vi "Obtain Request Events.vi"(8 "error in (no error)":errorcluster, 10 "Create New? (F)":bool) -> (0 "error out":errorcluster, 2 "Panther Dashboard Request Events":T1)   [LabVIEW 2023, in "Panther Dashboard.lvlib"]
doc: "This VI Obtains/Creates the Requests events that will be used for other modules to communicate with the module that owns this VI. These Requests events will be accessed only via Public API methods for this module.\n\n<b>NOTE</b>: The contents of this VI are automatically generated and modified by the <b>Tools > Delacor > DQMH</b> utilities. Consider using those utilities instead of making your own modifications to this VI.\n_____\nBased on DQMH Project Template 6.1.0.94."
uses:
  Panther Dashboard.lvlib
  Request Events--cluster.ctl
  Stop Argument--cluster.ctl
  Show Panel Argument--cluster.ctl
  Hide Panel Argument--cluster.ctl
  Get Module Execution Status Argument--cluster.ctl
  Show Diagram Argument--cluster.ctl
  Scan DQMH Modules Argument--cluster.ctl
  Tree DQMH Selection Argument--cluster.ctl
  Open Module API Tester Argument--cluster.ctl
  Execute Default Event Request Argument--cluster.ctl
  Expand Results Argument--cluster.ctl
  Launch DQMH Scripting Tools Argument--cluster.ctl
  DQMH Tools Menu--enum.ctl
  Generate Project Documentation Argument--cluster.ctl
  Set App Theme Argument--cluster.ctl
  Show About Argument--cluster.ctl
  Update Module ID Argument--cluster.ctl
  Save Library Description Argument--cluster.ctl
  Save VI Description Argument--cluster.ctl
  Open Documentation Argument--cluster.ctl
  Save Project Documentation Argument--cluster.ctl
  Register controls Mouse Enter Argument--cluster.ctl
  Save Module Spec Argument--cluster.ctl
panel:
  # "NOTE: The contents of this VI are automatically generated and modified by the Tools > Delacor > DQMH utilities. Consider using those utilities instead of making your own modifications to this VI."
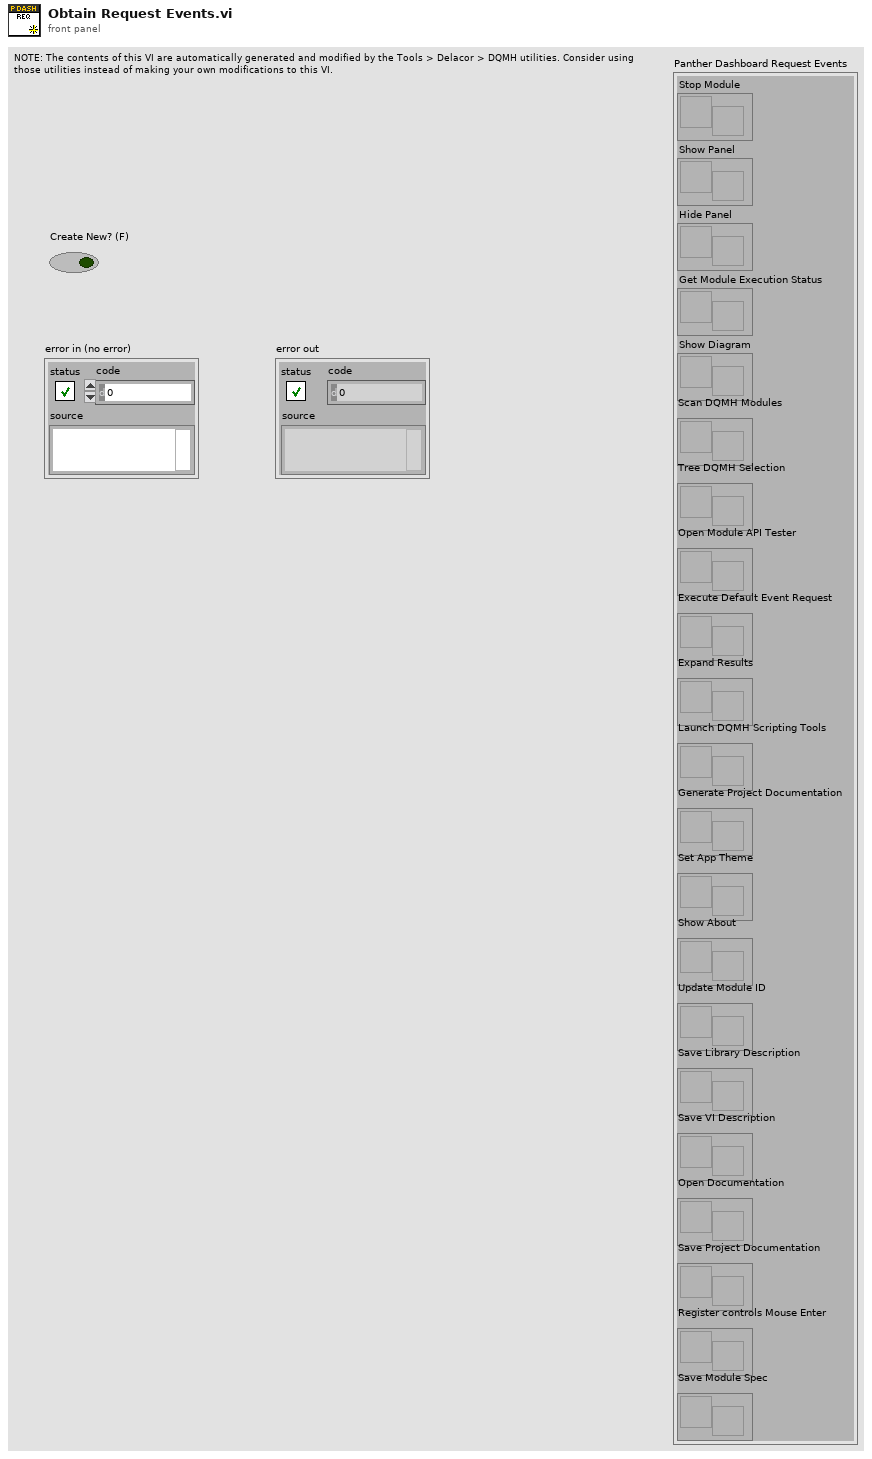
[diagram p1: front panel]
types:
  T1 = typedef "Panther Dashboard.lvlib/Request Events--cluster.ctl" = cluster{"Stop Module":refnum<user-event>, "Show Panel":refnum<user-event>, "Hide Panel":refnum<user-event>, "Get Module Execution Status":refnum<user-event>, "Show Diagram":refnum<user-event>, "Scan DQMH Modules":refnum<user-event>, "Tree DQMH Selection":refnum<user-event>, "Open Module API Tester":refnum<user-event>, "Execute Default Event Request":refnum<user-event>, "Expand Results":refnum<user-event>, "Launch DQMH Scripting Tools":refnum<user-event>, "Generate Project Documentation":refnum<user-event>, "Set App Theme":refnum<user-event>, "Show About":refnum<user-event>, "Update Module ID":refnum<user-event>, "Save Library Description":refnum<user-event>, "Save VI Description":refnum<user-event>, "Open Documentation":refnum<user-event>, "Save Project Documentation":refnum<user-event>, "Register controls Mouse Enter":refnum<user-event>, "Save Module Spec":refnum<user-event>}
  T2 = typedef "Panther Dashboard.lvlib/Save Module Spec Argument--cluster.ctl" = cluster{"Boolean":bool}
  T3 = typedef "Panther Dashboard.lvlib/Register controls Mouse Enter Argument--cluster.ctl" = cluster{"Boolean":bool}
  T4 = typedef "Panther Dashboard.lvlib/Save Project Documentation Argument--cluster.ctl" = cluster{"Project Description":string}
  T5 = typedef "Panther Dashboard.lvlib/Open Documentation Argument--cluster.ctl" = cluster{"Boolean":bool}
  T6 = typedef "Panther Dashboard.lvlib/Save VI Description Argument--cluster.ctl" = cluster{"VI Description":string}
  T7 = typedef "Panther Dashboard.lvlib/Save Library Description Argument--cluster.ctl" = cluster{"Library Description":string}
  T8 = typedef "Panther Dashboard.lvlib/Update Module ID Argument--cluster.ctl" = cluster{"New ID":i32}
  T9 = typedef "Panther Dashboard.lvlib/Show About Argument--cluster.ctl" = cluster{"Boolean":bool}
  T10 = typedef "Panther Dashboard.lvlib/Set App Theme Argument--cluster.ctl" = cluster{"Theme":bool}
  T11 = typedef "Panther Dashboard.lvlib/Generate Project Documentation Argument--cluster.ctl" = cluster{"Boolean":bool}
  T12 = typedef "Panther Dashboard.lvlib/Launch DQMH Scripting Tools Argument--cluster.ctl" = cluster{"Scripting Tool":T13}
  T13 = typedef "Panther Dashboard.lvlib/DQMH Tools Menu--enum.ctl" = enum16{"Create New DQMH Event", "Remove DQMH Event", "Convert DQMH Event", "Rename DQMH Event", "Add New DQMH Module", "Create RT Tester", "Rename DQMH Module", "Validate DQMH Module", "Create DQMH Module Template", "New DQMH  Unit Test", "Add Helper Loop to DQMH Module"}
  T14 = typedef "Panther Dashboard.lvlib/Expand Results Argument--cluster.ctl" = cluster{"Expand?":bool}
  T15 = typedef "Panther Dashboard.lvlib/Execute Default Event Request Argument--cluster.ctl" = cluster{"Event Name":string}
  T16 = typedef "Panther Dashboard.lvlib/Open Module API Tester Argument--cluster.ctl" = cluster{"Boolean":bool}
  T17 = typedef "Panther Dashboard.lvlib/Tree DQMH Selection Argument--cluster.ctl" = cluster{"Tree DQMH Sel":string}
  T18 = typedef "Panther Dashboard.lvlib/Scan DQMH Modules Argument--cluster.ctl" = cluster{"Include Dependencies":bool, "Scan All":bool, "Project":string, "Target":string}
  T19 = typedef "Panther Dashboard.lvlib/Hide Panel Argument--cluster.ctl" = cluster{"Hide Panel?":bool}
  T20 = typedef "Panther Dashboard.lvlib/Show Panel Argument--cluster.ctl" = cluster{"Show Panel?":bool}
  T21 = typedef "Panther Dashboard.lvlib/Show Diagram Argument--cluster.ctl" = cluster{"Debug?":bool}
  T22 = typedef "Panther Dashboard.lvlib/Get Module Execution Status Argument--cluster.ctl" = cluster{"Running?":bool}
  T23 = typedef "Panther Dashboard.lvlib/Stop Argument--cluster.ctl" = cluster{"Origin":string, "Exit via Stop Module Req?":bool, "Wait for Module to stop?":bool}
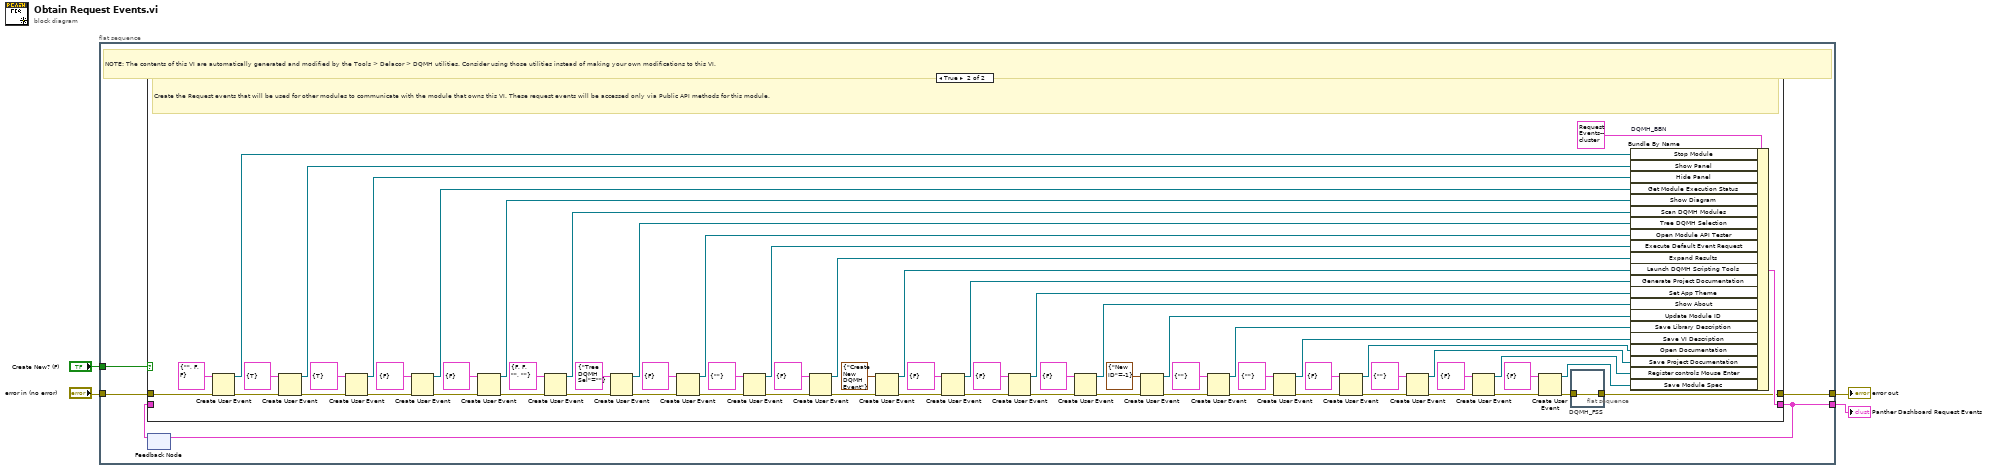
[diagram p0: block diagram]
diagram:
  n1 = flat-sequence {
    tunnel: [w9] -> w4
    tunnel: "error in (no error)" -> [w8]
    tunnel: [w6] -> w2
    tunnel: "Create New? (F)" -> [w5]
    frame #0 {
      # "NOTE: The contents of this VI are automatically generated and modified by the Tools > Delacor > DQMH utilities. Consider using those utilities instead of making your own modifications to this VI."
      n2 = feedback #1() -> (w7:T1)  [unwired: 1 in]
      n3 = case shown="True" w5 {
        tunnel: [w10 w68] -> w9
        tunnel: w8 -> [w10 w78]
        tunnel: [w11 w75] -> w6
        tunnel: w7 -> [w11 _]
        frame False {
          # "Obtain the Request events that were created in a previous call to this VI."
        }
        frame True {
          # "Create the Request events that will be used for other modules to communicate with the module that owns this VI. These request events will be accessed only via Public API methods for this module."
          n4 = Create User Event(user event datatype=T23 {"Origin"="", "Exit via Stop Module Req?"=FALSE, "Wait for Module to stop?"=FALSE} ("Stop Argument"), error in=w78) -> (user event=w76:refnum<user-event>, error out=w73:errorcluster)
          n5 = Create User Event(user event datatype=T20 {"Show Panel?"=TRUE} ("Show Panel Argument"), error in=w73) -> (user event=w72:refnum<user-event>, error out=w71:errorcluster)
          n6 = Create User Event(user event datatype=T19 {"Hide Panel?"=TRUE} ("Hide Panel Argument"), error in=w71) -> (user event=w70:refnum<user-event>, error out=w69:errorcluster)
          n7 = Create User Event(user event datatype=T22 {"Running?"=FALSE} ("Get Module Execution Status Argument"), error in=w69) -> (user event=w66:refnum<user-event>, error out=w67:errorcluster)
          n8 = Create User Event(user event datatype=T21 {"Debug?"=FALSE} ("Show Diagram Argument"), error in=w67) -> (user event=w63:refnum<user-event>, error out=w64:errorcluster)
          n9 = Create User Event(user event datatype=T18 {"Include Dependencies"=FALSE, "Scan All"=FALSE, "Project"="", "Target"=""} ("Scan DQMH Modules Argument"), error in=w64) -> (user event=w58:refnum<user-event>, error out=w59:errorcluster)
          n10 = Create User Event(user event datatype=T17 {"Tree DQMH Sel"=""} ("Tree DQMH Selection Argument"), error in=w59) -> (user event=w55:refnum<user-event>, error out=w56:errorcluster)
          n11 = Create User Event(user event datatype=T16 {"Boolean"=FALSE} ("Open Module API Tester Argument"), error in=w56) -> (user event=w52:refnum<user-event>, error out=w53:errorcluster)
          n12 = Create User Event(user event datatype=T15 {"Event Name"=""} ("Execute Default Event Request Argument"), error in=w53) -> (user event=w49:refnum<user-event>, error out=w50:errorcluster)
          n13 = Create User Event(user event datatype=T14 {"Expand?"=FALSE} ("Expand or Close Argument"), error in=w50) -> (user event=w46:refnum<user-event>, error out=w47:errorcluster)
          n14 = Create User Event(user event datatype=T12 {"Scripting Tool"=enum."Create New DQMH Event"} ("Launch DQMH Scripting Tools Argument"), error in=w47) -> (user event=w43:refnum<user-event>, error out=w44:errorcluster)
          n15 = Create User Event(user event datatype=T11 {"Boolean"=FALSE} ("Generate Project Documentation Argument"), error in=w44) -> (user event=w40:refnum<user-event>, error out=w41:errorcluster)
          n16 = Create User Event(user event datatype=T10 {"Theme"=FALSE} ("Set App Theme Argument"), error in=w41) -> (user event=w37:refnum<user-event>, error out=w38:errorcluster)
          n17 = Create User Event(user event datatype=T9 {"Boolean"=FALSE} ("Show About Argument"), error in=w38) -> (user event=w34:refnum<user-event>, error out=w35:errorcluster)
          n18 = Create User Event(user event datatype=T8 {"New ID"=-1} ("Update Module ID Argument"), error in=w35) -> (user event=w31:refnum<user-event>, error out=w32:errorcluster)
          n19 = Create User Event(user event datatype=T7 {"Library Description"=""} ("Save Library Description Argument"), error in=w32) -> (user event=w28:refnum<user-event>, error out=w29:errorcluster)
          n20 = Create User Event(user event datatype=T6 {"VI Description"=""} ("Save VI Description Argument"), error in=w29) -> (user event=w25:refnum<user-event>, error out=w26:errorcluster)
          n21 = Create User Event(user event datatype=T5 {"Boolean"=FALSE} ("Open Documentation Argument"), error in=w26) -> (user event=w22:refnum<user-event>, error out=w23:errorcluster)
          n22 = Create User Event(user event datatype=T4 {"Project Description"=""} ("Save Project Documentation Argument"), error in=w23) -> (user event=w19:refnum<user-event>, error out=w20:errorcluster)
          n23 = Create User Event(user event datatype=T3 {"Boolean"=FALSE} ("Register controls Mouse Enter Argument"), error in=w20) -> (user event=w16:refnum<user-event>, error out=w17:errorcluster)
          n24 = Create User Event(user event datatype=T2 {"Boolean"=FALSE} ("Save Module Spec Argument"), error in=w17) -> (user event=w13:refnum<user-event>, error out=w14:errorcluster)
          n25 = flat-sequence "DQMH_FSS" {
            tunnel: w14 -> [w79]
            tunnel: [w79] -> w68
            frame #0 {
            }
          }
          n26 = Bundle By Name "DQMH_BBN"(cluster=T1 {"Stop Module"=refnum, "Show Panel"=refnum, "Hide Panel"=refnum, "Get Module Execution Status"=refnum, "Show Diagram"=refnum, "Scan DQMH Modules"=refnum, "Tree DQMH Selection"=refnum, "Open Module API Tester"=refnum, "Execute Default Event Request"=refnum, "Expand Results"=refnum, "Launch DQMH Scripting Tools"=refnum, "Generate Project Documentation"=refnum, "Set App Theme"=refnum, "Show About"=refnum, "Update Module ID"=refnum, "Save Library Description"=refnum, "Save VI Description"=refnum, "Open Documentation"=refnum, "Save Project Documentation"=refnum, "Register controls Mouse Enter"=refnum, "Save Module Spec"=refnum} ("output cluster"), "Stop Module"=w76, "Show Panel"=w72, "Hide Panel"=w70, "Get Module Execution Status"=w66, "Show Diagram"=w63, "Scan DQMH Modules"=w58, "Tree DQMH Selection"=w55, "Open Module API Tester"=w52, "Execute Default Event Request"=w49, "Expand Results"=w46, "Launch DQMH Scripting Tools"=w43, "Generate Project Documentation"=w40, "Set App Theme"=w37, "Show About"=w34, "Update Module ID"=w31, "Save Library Description"=w28, "Save VI Description"=w25, "Open Documentation"=w22, "Save Project Documentation"=w19, "Register controls Mouse Enter"=w16, "Save Module Spec"=w13) -> (w75:T1)
        }
      }
      n27 = feedback-in #1(w6) -> ()
    }
  }
  "Panther Dashboard Request Events" <- w2
  "error out" <- w4
